vi "Error Message Code.vi"(7 "Enum":enum16{"Initial", "ErrorIn"}(ring)=enum."ErrorIn", 10 "SHBIndex":string, 11 "Error Code":i32=5000) -> (3 "Error Message":T1)   [LabVIEW 2019]
uses:
  LLB/Commonly VI/Main Glb.vi
  <vilib>/Utility/config.llb/Read Key (String).vi
  <vilib>/Utility/config.llb/NI_LVConfig.lvlib
  LLB/Commonly VI.lvlib
panel:
  out "Error Message array English 2":string[][](array[string])
  in  "Error Message array Chinese 6000-9006":string[][](array[string])
  in  "Error Message array Chinese 5045-6000":string[][](array[string])
  in  "Error Message array English":string[][](array[string])=[["5000", "Emergency Stop Error/ Check Emergency Stop Button"], ["5001", "Air Pressure Error/ Check whether air pressure is in standard range"], ["5002", "Motor control Error/ Check whether motion control card sets properly"], ["5003", ""], ["5004", "Motion Timeout/Check whether XY table is malfunction"], ["5005", "承載Stack (A-1) 側上下軸Servo Ready逾時/請確認承載Stack (A-1) 側上下軸驅動器狀態"], ["5006", "承載Stack (A-2 側上下軸Servo Ready逾時/請確認承載Stack (A-2) 側上下軸驅動器狀態"], ["5007", "承載Stack (B-1) 側上下軸Servo Ready逾時/請確認承載Stack (B-1) 側上下軸驅動器狀態"], ["5008", "承載Stack (B-2) 側上下軸Servo Ready逾時/請確認承載Stack (B-2) 側上下軸驅動器狀態"], ["5009", "承載Loader (A) 移載軸Servo Ready逾時/請確認承載Loader (A) 移載軸驅動器狀態"], ["5010", "承載Loader (B) 移載軸Servo Ready逾時/請確認承載Loader (B) 移載軸驅動器狀態"], ["5011", "Stack傳送帶軸Servo Ready逾時/請確認Stack傳送帶軸驅動器狀態"], ["5012", "None"], ["5013", "前定位傳送帶軸Servo Ready逾時/請確認前定位傳送帶軸驅動器狀態,Power ON是否正確按下"], ["5014", "ÀË´ú¶Ç°e±a(1)¶bServo Ready¹O®É/½Ð½T»{ÀË´ú¶Ç°e±a(1)¶bÅX°Ê¾¹ª¬ºA,Power ON¬O§_¥¿½T«ö¤U"], ["5015", "ÀË´ú¶Ç°e±a(2)¶bServo Ready¹O®É/½Ð½T»{ÀË´ú¶Ç°e±a(2)¶bÅX°Ê¾¹ª¬ºA,Power ON¬O§_¥¿½T«ö¤U"], ["5016", " ÀË´ú¶Ç°e±a(3)¶bServo Ready¹O®É/½Ð½T»{ÀË´ú¶Ç°e±a(3)¶bÅX°Ê¾¹ª¬ºA,Power ON¬O§_¥¿½T«ö¤U"], ["5017", "後定位傳送帶軸Servo Ready逾時/請確認後定位傳送帶軸驅動器狀態,Power ON是否正確按下"], ["5018", "分類傳送帶軸Servo Ready逾時/請確認分類傳送帶軸驅動器狀態,Power ON是否正確按下"], ["5019", "分類區(1)移載軸Servo Ready逾時/請確認分類區(1)移載軸驅動器狀態,Power ON是否正確按下"], ["5020", "分類區(2)移載軸Servo Ready逾時/請確認分類區(2)移載軸驅動器狀態,Power ON是否正確按下"], ["5021", "分類區(3)移載軸Servo Ready逾時/請確認分類區(3)移載軸驅動器狀態,Power ON是否正確按下"], ["5022", "分類區(4)移載軸Servo Ready逾時/請確認分類區(4)移載軸驅動器狀態,Power ON是否正確按下"], ["5023", "分類區(5)移載軸Servo Ready逾時/請確認分類區(5)移載軸驅動器狀態,Power ON是否正確按下"], ["5024", "分類區(6)移載軸Servo Ready逾時/請確認分類區(6)移載軸驅動器狀態,Power ON是否正確按下"], ["5025", "承載Stack (A-1) 側上下軸移動逾時/請確認承載Stack (A-1) 側上下軸狀態,Power ON是否正確按下"], ["5026", "承載Stack (A-2) 側上下軸移動逾時/請確認承載Stack (A-2) 側上下軸狀態,Power ON是否正確按下"], ["5027", "承載Stack (B-1) 側上下軸移動逾時/請確認承載Stack (B-1) 側上下軸狀態,Power ON是否正確按下"], ["5028", "承載Stack (B-2) 側上下軸移動逾時/請確認承載Stack (B-2) 側上下軸狀態,Power ON是否正確按下"], ["5029", "承載Loader (A) 移載軸移動逾時/請確認承載Loader (A) 移載軸狀態,Power ON是否正確按下"], ["5030", "承載Loader (B) 移載軸移動逾時/請確認承載Loader (B) 移載軸狀態,Power ON是否正確按下"], ["5031", "Stack傳送帶軸移動逾時/請確認Stack傳送帶軸狀態,Power ON是否正確按下"], ["5032", "None"], ["5033", "前定位傳送帶軸移動逾時/請確認前定位傳送帶軸狀態,Power ON是否正確按下"], ["5034", "檢測傳送帶(1)軸移動逾時/請確認檢測傳送帶(1)軸狀態,Power ON是否正確按下"], ["5035", "檢測傳送帶(2)軸移動逾時/請確認檢測傳送帶(2軸狀態,Power ON是否正確按下"], ["5036", "檢測傳送帶(3)軸移動逾時/請確認檢測傳送帶(3)軸狀態,Power ON是否正確按下"], ["5037", "後定位傳送帶軸移動逾時/請確認後定位傳送帶軸狀態,Power ON是否正確按下"], ["5038", "分類傳送帶軸移動逾時/請確認分類傳送帶軸狀態,Power ON是否正確按下"], ["5039", "分類區(1)移載軸移動逾時/請確認分類區(1)移載軸狀態,Power ON是否正確按下"], ["5040", "分類區(2)移載軸移動逾時/請確認分類區(2)移載軸狀態,Power ON是否正確按下"], ["5041", "分類區(3)移載軸移動逾時/請確認分類區(3)移載軸狀態,Power ON是否正確按下"], ["5042", "分類區(4)移載軸移動逾時/請確認分類區(4)移載軸狀態,Power ON是否正確按下"], ["5043", "分類區(5)移載軸移動逾時/請確認分類區(5)移載軸狀態,Power ON是否正確按下"], ["5044", "分類區(6)移載軸移動逾時/請確認分類區(6)移載軸狀態,Power ON是否正確按下"], ["5045", "Emergency Stop ON Timeout/ Check Emergency Stop button"], ["5046", "機台啟動/復歸開關ON逾時/請確認機台啟動/復歸開關是否異常"], ["5047", "Air Pressure ON Timeout/ Check whether air pressure is in standard range"], ["5048", "Door Opened/ Make sure doors are all closed"], ["5049", "Optical grating Error/ Make sure no objects are in Optical grating"], ["5050", "Feeder In Auto Signal Timeout/ Check whether feeder In is in auto mode"], ["5051", "Feeder In Finish Signal Timeout"], ["5052", "Feeder In Tray Ready Signal Timeout/ Check whether feeder in works properly"], ["5053", "Feeder Out Auto Signal Timeout/ Check whether feeder Out is in auto mode"], ["5054", "Feeder Out Finish Signal Timeout"], ["5055", "Feeder Out Tray Ready Signal Timeout/ Check whether feeder Out works properly"], ["5056", "進料機B Ready檢知ON逾時/請確認進料機B Ready檢知是否正常"], ["5057", "進料機B ALARM檢知ON逾時/請確認進料機B ALARM檢知是否正常"], ["5058", "進料機B 通知滑台可吸料檢知ON逾時/請確認進料機B 通知滑台可吸料檢知是否正常"], ["5059", "良品機B Ready檢知ON逾時/請確認良品機B Ready檢知是否正常"], ["5060", "良品機B ALARM檢知ON逾時/請確認良品機B ALARM檢知是否正常"], ["5061", "良品機B 通知滑台可吸料檢知ON逾時/請確認良品機B 通知滑台可吸料檢知是否正常"], ["5062", "Nozzle 1 Vacuum Check On Timeout/ Check Nozzle 1"], ["5063", "Nozzle 2 Vacuum Check On Timeout/ Check Nozzle 2"], ["5064", "吸嘴3真空檢知ON逾時/請確認吸嘴3真空檢知異常情形"], ["5065", "吸嘴4真空檢知ON逾時/請確認吸嘴4真空檢知異常情形"], ["5066", "Tool 1 Position On Timeout/ Check whether tool 1 is malfunction"], ["5067", "Tool 2 Position On Timeout/ Check whether tool 2 is malfunction"], ["5068", "雷射測距HIGH 判斷ON逾時/請確認雷射測距HIGH是否正常"], ["5069", "雷射測距LOW判斷ON逾時/請確認雷射測距LOW是否正常"], ["5070", "雷射測距GO判斷ON逾時/請確認雷射測距GO是否正常"], ["5071", "雷射測距警報ON逾時/請確認雷射測距警報是否正常"], ["5072", "Emergency Stop Off Timeout/ Check Emergency Stop button"], ["5073", "機台電源啟動開關OFF逾時/請確認機台電源是否異常"], ["5074", "Air Pressure Off Timeout/ Check whether air pressure is in standard "], ["5075", "Door Opened/ Make sure doors are all closed"], ["5076", "Optical grating Error/ Make sure no objects are in Optical grating"], ["5077", "Feeder In Auto Signal Off Timeout/ Check whether feeder In is in auto mode"], ["5078", "Feeder In Finish Signal Off Timeout"], ["5079", "Feeder In Tray Ready Signal OffTimeout/ Check whether feeder in works properly"], ["5080", "Feeder Out Auto Signal Off Timeout/ Check whether feeder Out is in auto mode"], ["5081", "Feeder Out Finish Signal Off Timeout"], ["5082", "Feeder Out Tray Ready Signal Timeout/ Check whether feeder Out works properly"], ["5083", "進料機B Ready檢知OFF逾時/請確認進料機B Ready檢知是否正常"], ["5084", "進料機B ALARM檢知OFF逾時/請確認進料機B ALARM檢知是否正常"], ["5085", "進料機B 通知滑台可吸料檢知OFF逾時/請確認進料機B 通知滑台可吸料檢知是否正常"], ["5086", "良品機B Ready檢知OFF逾時/請確認良品機B Ready檢知是否正常"], ["5087", "良品機B ALARM檢知OFF逾時/請確認良品機B ALARM檢知是否正常"], ["5088", "良品機B 通知滑台可吸料檢知OFF逾時/請確認良品機B 通知滑台可吸料檢知是否正常"], ["5089", "Nozzle 1 Vacuum Check Off Timeout/ Check Nozzle 1"], ["5090", "Nozzle 2 Vacuum Check Off Timeout/ Check Nozzle 2"], ["5091", "吸嘴3真空檢知OFF逾時/請確認吸嘴3真空檢知異常情形"], ["5092", "吸嘴4真空檢知OFF逾時/請確認吸嘴4真空檢知異常情形"], ["5093", "Tool 1 Position Off Timeout/ Check whether tool 1 is malfunction"], ["5094", "Tool 2 Position Off Timeout/ Check whether tool 2 is malfunction"], ["5095", "雷射測距HIGH 判斷OFF逾時/請確認雷射測距HIGH是否正常"], ["5096", "雷射測距LOW判斷OFF逾時/請確認雷射測距LOW是否正常"], ["5097", "雷射測距GO判斷OFF逾時/請確認雷射測距GO是否正常"], ["5098", "雷射測距警報OFF逾時/請確認雷射測距警報是否正常"], ["", ""], ["6000", "Dut didn't place properly/ Check Dut"], ["6001", "Fail Tray Full/ Replace with a empty Fail Tray"], ["6002", "Dut Scan Fail/ Check Dut"], ["6003", "Down Vision Out of Range/ Check Dut"], ["6004", "SHB 1 Back Sensor Check ON Error"], ["6005", "SHB 2 Back Sensor Check ON Error"], ["6006", "SHB 3 Back Sensor Check ON Error"], ["6007", "SHB 4 Back Sensor Check ON Error"], ["7000", "SHB  Not Feedback Start Test OK"], ["7001", "SHB 1 Not Feedback Start Test OK"], ["7002", "SHB 2 Not Feedback Start Test OK"], ["7003", "SHB 3 Not Feedback Start Test OK"], ["7004", "SHB 4 Not Feedback Start Test OK"], ["7101", "SHB 1 Command Type Error"], ["7102", "SHB 2 Command Type Error"], ["7103", "SHB 3 Command Type Error"], ["7104", "SHB 4 Command Type Error"], ["7105", "SHB 1 Detection Error"], ["7106", "SHB 2 Detection Error"], ["7107", "SHB 3 Detection Error"], ["7108", "SHB 4 Detection Error"], ["8001", "Change DUT Tray"], ["8002", "Change PASS Tray"], ["8003", "Change Fail Tray"], ["8004", "Check DUT Tray"], ["8005", "Check PASS Tray"], ["9001", "Dn Vision No Found DUT"], ["9002", "Dn Vision Angle Out of Range"], ["9003", "Dn Vision XY Out of Range"], ["9006", "RobotTimeOut"]]
  in  "Error Message array Chinese (原始資料)":string[][](array[string])
  # "5000-5002 emergency\n5004-5043 general\n5045-5071 I/O On time out\n5072-5098 I/O Off time out\n6000-          Motion Error\n7000            SHB Timeout* \n7001-7100 SHBTimeout\n7101-7200 SHB Error\n8001-8005 TRAY\n9001-9005 Vision\n9006            RobotTimeOut"
  # "7000: 不明錯誤，隔離箱Index 被寫0"
  # "記得離開要Make Default 存檔"
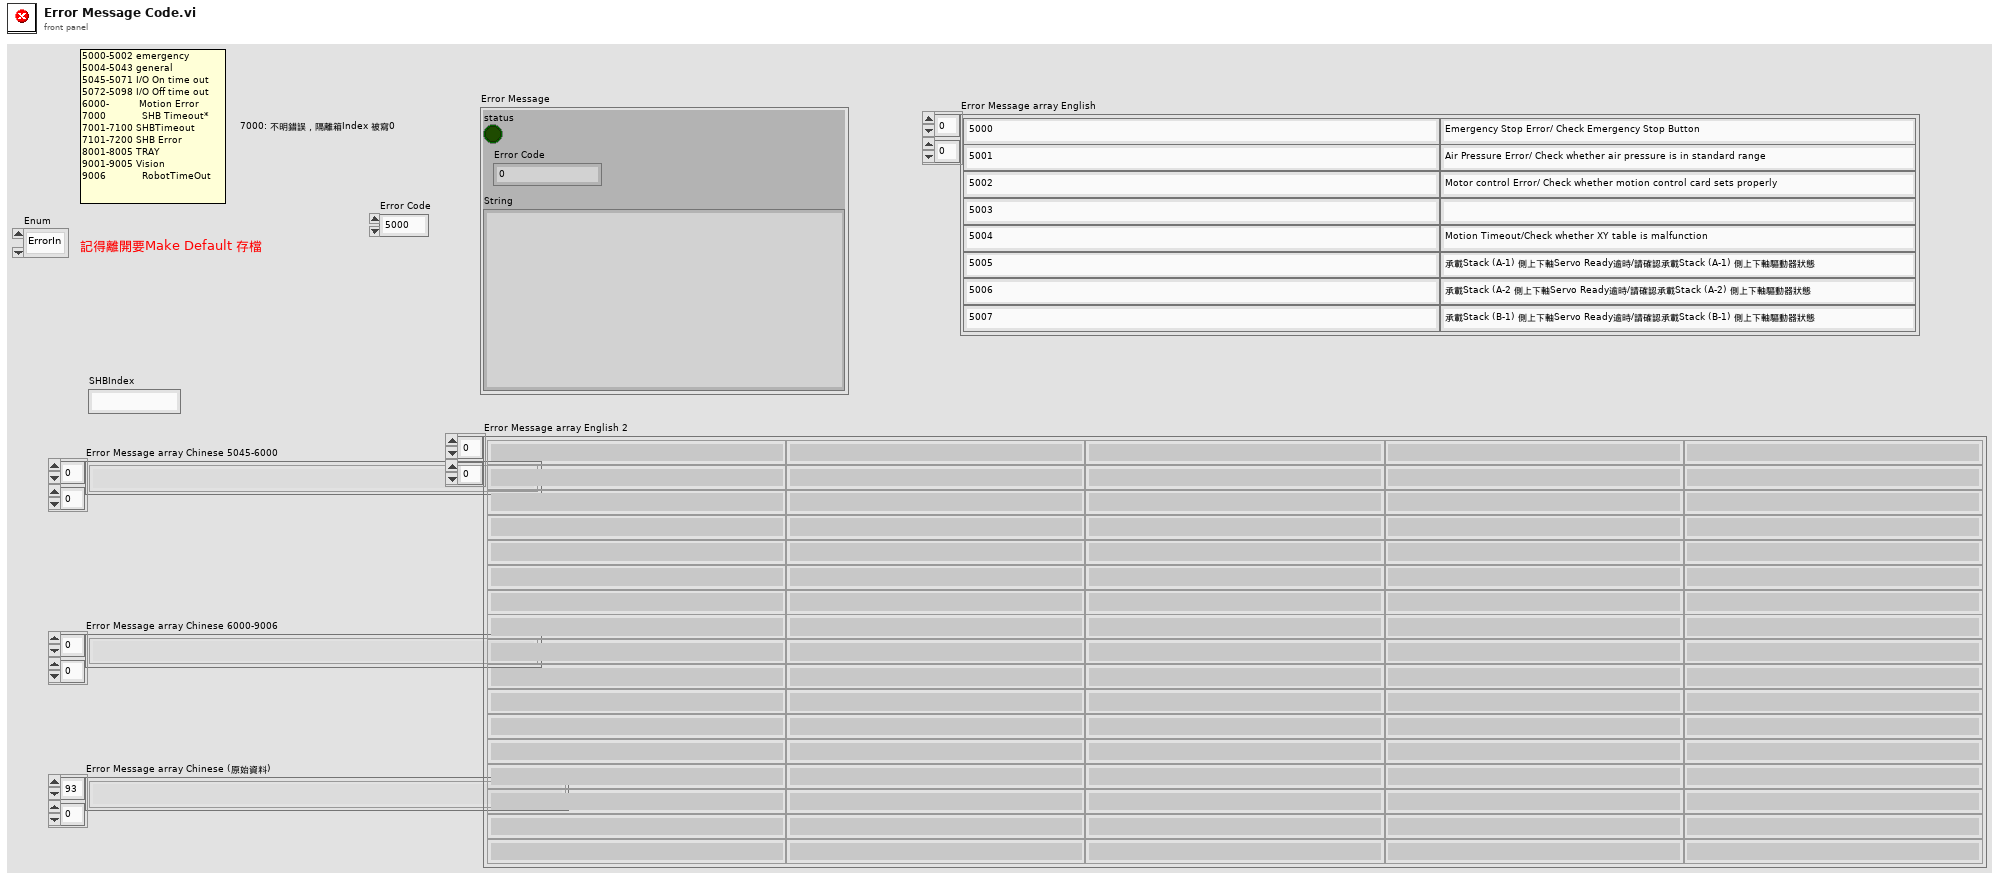
[diagram p1: front panel]
types:
  T1 = cluster{"status":bool, "Error Code":i32, "String":string}
  T2 = enum16{"open", "replace", "create", "open or create", "replace or create", "replace or create with confirmation"}
  T3 = typedef "NI_LVConfig.lvlib/Config Data RefNum.ctl" = refnum<k1>
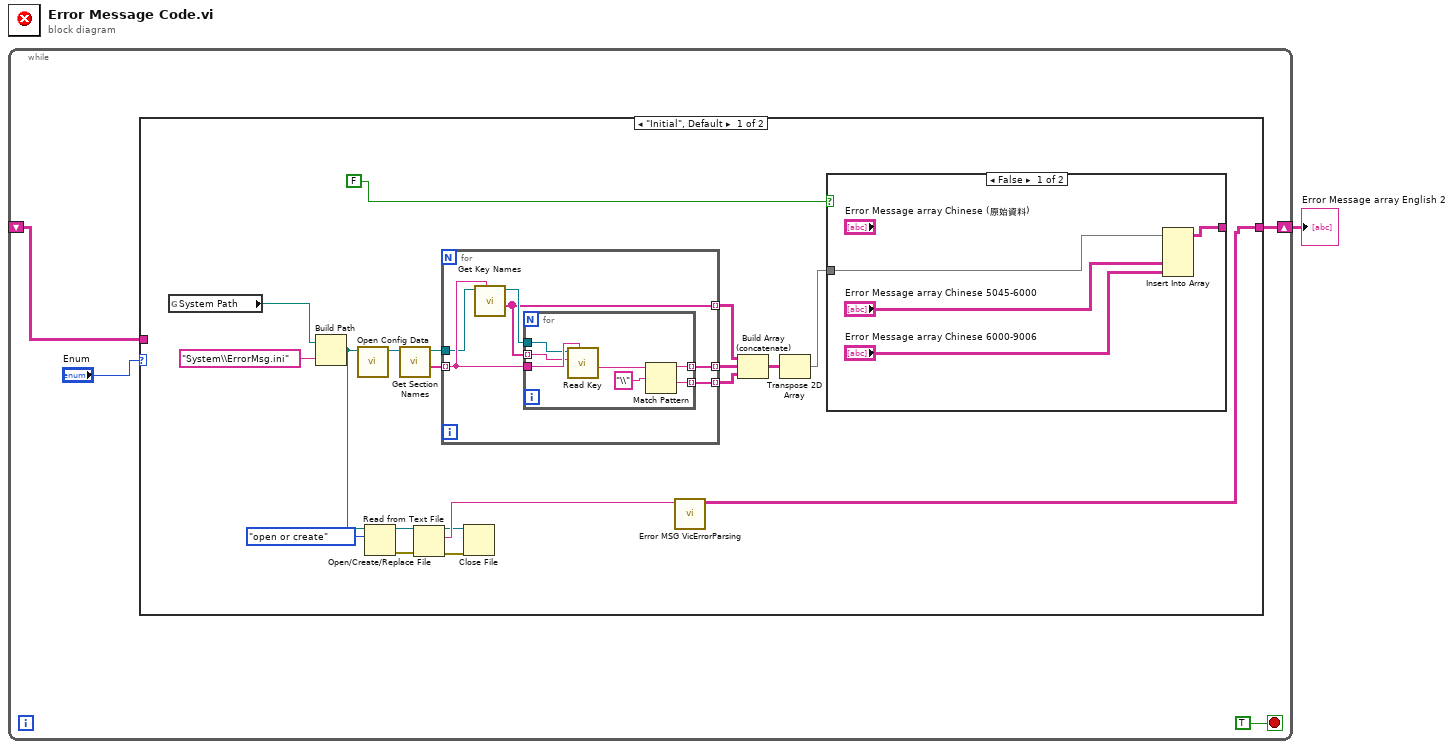
[diagram p0: block diagram]
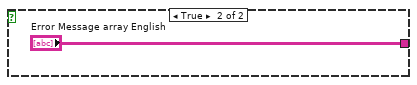
[diagram p2: hidden frame]
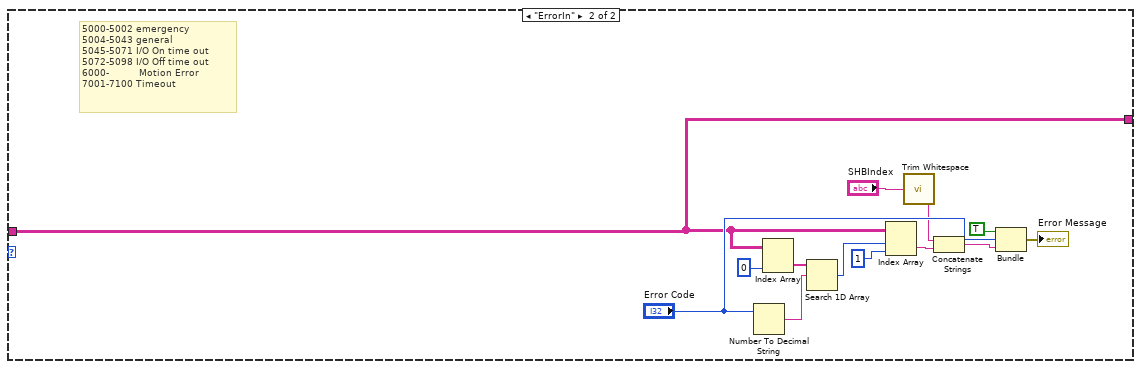
[diagram p3: hidden frame]
diagram:
  n1 = while {
    shift-right: [w4] -> w1
    shift-left: _ -> [w3]
    stop <- TRUE stop-if-true
    n2 = case shown="\"Initial\", Default" "Enum" {
      tunnel: [w14 w48] -> w4
      tunnel: w3 -> [_ w48]
      frame "Initial", Default {
        n3 = global read "Main Glb.vi" "System Path"() -> (w6:path)
        n4 = Build Path(base path=w6, name or relative path="System\\ErrorMsg.ini") -> (appended path=w13:path)
        n5 = call <vilib>:"Open Config Data.vi"("configuration file path"=w13) -> ("refnum"=w23:T3)  [unwired: 8 in, 2 out]
        n6 = Open/Create/Replace File(file path (use dialog)=w13, operation (0:open)=T2."open or create") -> (refnum out=w11:refnum<file>, error out=w12:errorcluster)  [unwired: 4 in, 1 out]
        n7 = call <vilib>:"Get Section Names.vi"("refnum"=w23) -> ("section names"=w19:string[], "refnum out"=w22:T3)  [unwired: 8 in, 1 out]
        n8 = Read from Text File(file (use dialog)=w11, error in=w12) -> (refnum out=w8:refnum<file>, text=w9:string, error out=w7:errorcluster)  [unwired: 2 in, 1 out]
        n9 = for {
          tunnel: w19 -> [w30] mode=indexing
          tunnel: w22 -> [w29]
          tunnel: [w27] -> w21 mode=indexing
          tunnel: [w26] -> w18 mode=indexing
          tunnel: [w25] -> w17 mode=indexing
          n10 = call <vilib>:"Get Key Names.vi"("section"=w30, "refnum"=w29) -> ("key names"=w26:string[], "refnum out"=w28:T3)  [unwired: 6 in, 2 out]
          n11 = for {
            tunnel: w30 -> [w37]
            tunnel: w26 -> [w36] mode=indexing
            tunnel: w28 -> [w35]
            tunnel: [w32] -> w27 mode=indexing
            tunnel: [w31] -> w25 mode=indexing
            n12 = call-poly <vilib>:"Read Key.vi"("section"=w37, "key"=w36, "refnum"=w35) -> ("value"=w34:string)  [unwired: 5 in, 3 out]
            n13 = Match Pattern(string=w34, regular expression="\\") -> (before substring=w32:string, after substring=w31:string)  [unwired: 1 in, 2 out]
          }
        }
        n14 = Close File(refnum=w8, error in=w7) -> ()  [unwired: 2 out]
        n15 = call "Error MSG VicErrorParsing.vi"("WrrmsgIn"=w9) -> ("MsgOut"=w14:string[][])  [unwired: 10 in]
        n16 = Build Array (concatenate)(w18, w21, w17) -> (w20:string[][])
        n17 = Transpose 2D Array(2D array=w20) -> (transposed array=w16:string[][])
        n18 = case shown="False" FALSE {
          tunnel: [w39 "Error Message array English"] -> _
          tunnel: w16 -> [w38 _]
          frame False {
            n19 = Insert Into Array(array=w38, new element #1="Error Message array Chinese 5045-6000", new element #2="Error Message array Chinese 6000-9006") -> (w39:string[][])  [unwired: 2 in]
          }
          frame True {
          }
        }
      }
      frame "ErrorIn" {
        # "5000-5002 emergency\n5004-5043 general\n5045-5071 I/O On time out\n5072-5098 I/O Off time out\n6000-          Motion Error\n7001-7100 Timeout"
        n20 = Number To Decimal String(number="Error Code") -> (decimal integer string=w53:string)  [unwired: 1 in]
        n21 = Index Array(array=w48, index (col)=0 ("disabled index (col)")) -> (element=w51:string[])  [unwired: 1 in]
        n22 = Search 1D Array(1D array=w51, element=w53) -> (index of element=w43:i32)  [unwired: 1 in]
        n23 = Index Array(array=w48, index (row)=w43, index (col)=1 ("disabled index (col)")) -> (element=w47:string)
        n24 = call <vilib>:"Trim Whitespace.vi"("string"="SHBIndex") -> ("trimmed string"=w44:string)  [unwired: 1 in]
        n25 = Concatenate Strings(w44, w47) -> (w46:string)
        n26 = Bundle("status"=TRUE, "Error Code"="Error Code", w46) -> (→"Error Message":cluster{"status":bool, "Error Code":i32, string})  [unwired: 1 in]
      }
    }
  }
  "Error Message array English 2" <- w1
